vi "Delete Data (Entire Stat Page).vi"(0 "Filepath":path, 11 "Error In":errorcluster) -> (15 "Error Out":errorcluster)   [LabVIEW 2013]
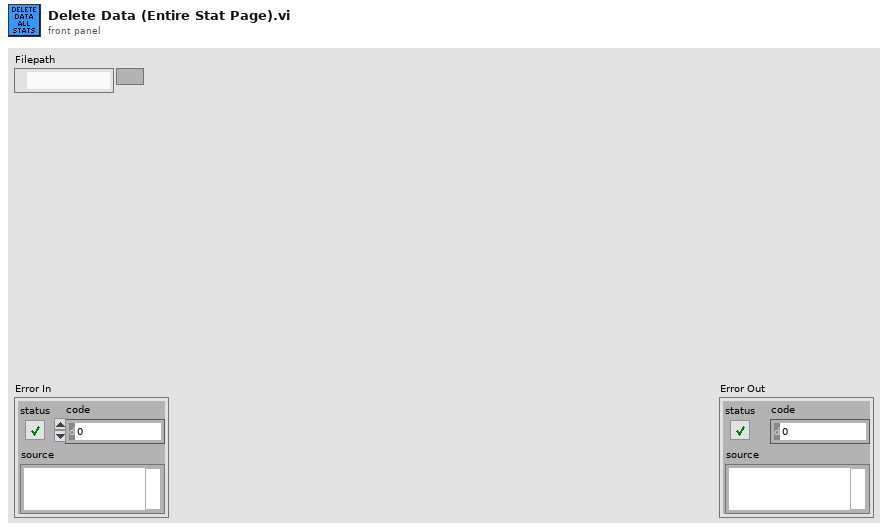
[diagram p1: front panel]
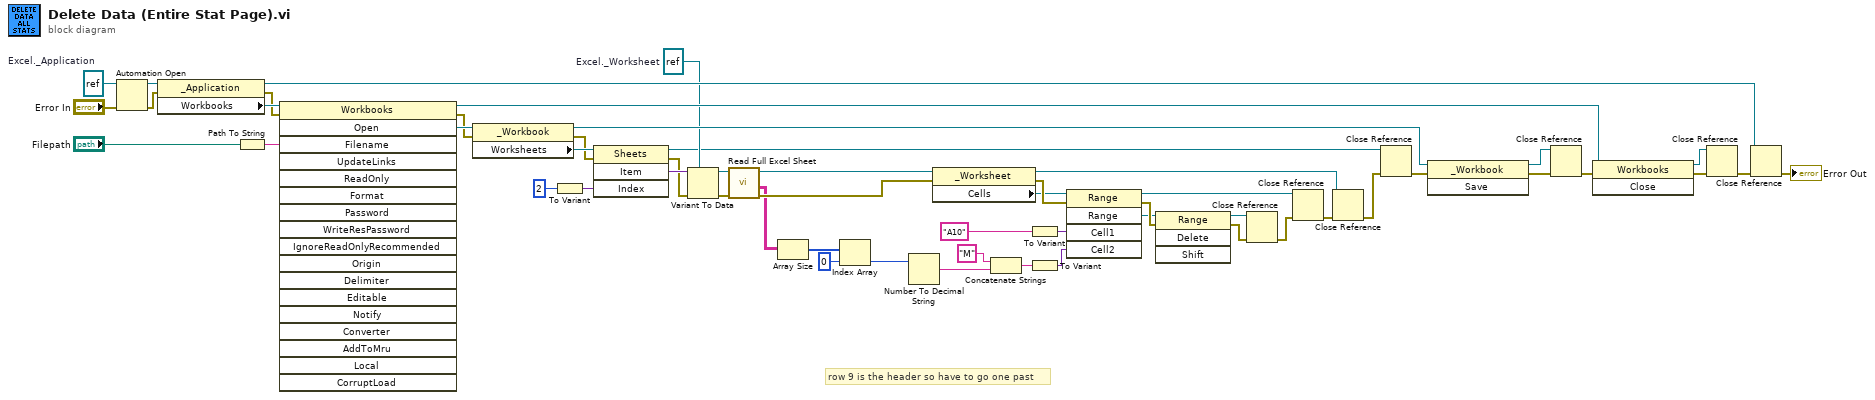
[diagram p0: block diagram]
diagram:
  w18 = refnum<k7> refnum  # Excel._Worksheet
  w51 = refnum<k7> refnum  # Excel._Application
  # "row 9 is the header so have to go one past"
  n1 = Automation Open(error in (no error)="Error In", Automation Refnum=w51) -> (Automation Refnum=w52:refnum<k7>, error out=w53:errorcluster)  [unwired: 2 in]
  n2 = property class="_Application"(reference=w52, error in=w53) -> (reference out=w44:refnum<k7>, error out=w45:errorcluster, "Workbooks"=w54:refnum<k7>)
  n3 = Path To String(path="Filepath") -> (string=w41:string)
  n4 = invoke class="Workbooks" method="Open"(reference=w54, error in=w45, "Filename"=w41) -> (reference out=w48:refnum<k7>, error out=w43:errorcluster, "Open"=w50:refnum<k7>)  [unwired: 15 in, 15 out]
  n5 = property class="_Workbook"(reference=w50, error in=w43) -> (reference out=w37:refnum<k7>, error out=w12:errorcluster, "Worksheets"=w13:refnum<k7>)
  n6 = To Variant(anything=2) -> (Variant=w19:variant)
  n7 = invoke class="Sheets" method="Item"(reference=w13, error in=w12, "Index"=w19) -> (reference out=w17:refnum<k7>, error out=w16:errorcluster, "Item"=w20:variant)  [unwired: 1 in, 1 out]
  n8 = Variant To Data(error in=w16, type=w18, Variant=w20) -> (data=w10:refnum<k7>, error out=w9:errorcluster)
  n9 = call "Read Full Excel Sheet.vi"("Error In"=w9, "Excel._Worksheet"=w10) -> ("Error Out"=w7:errorcluster, "Data"=w6:string[][], "Reference Out"=w8:refnum<k7>)  [unwired: 7 in]
  n10 = Array Size(array=w6) -> (size(s)=w5:i32[])
  n11 = Index Array(array=w5, index=0) -> (element=w3:i32)
  n12 = Number To Decimal String(number=w3) -> (decimal integer string=w14:string)  [unwired: 1 in]
  n13 = property class="_Worksheet"(reference=w8, error in=w7) -> (reference out=w22:refnum<k7>, error out=w26:errorcluster, "Cells"=w25:refnum<k7>)
  n14 = Concatenate Strings("M" ("ColumnIndex"), w14) -> (w32:string)
  n15 = To Variant(anything="A10" ("ColumnIndex")) -> (Variant=w24:variant)
  n16 = To Variant(anything=w32) -> (Variant=w28:variant)
  n17 = invoke class="Range" method="Range"(reference=w25, error in=w26, "Cell1"=w24, "Cell2"=w28) -> (reference out=w11:refnum<k7>, error out=w29:errorcluster, "Range"=w27:refnum<k7>)  [unwired: 1 in, 2 out]
  n18 = invoke class="Range" method="Delete"(reference=w27, error in=w29) -> (reference out=w30:refnum<k7>, error out=w31:errorcluster)  [unwired: 2 in, 2 out]
  n19 = Close Reference(reference=w30, error in (no error)=w31) -> (error out=w1:errorcluster)
  n20 = Close Reference(reference=w11, error in (no error)=w1) -> (error out=w21:errorcluster)
  n21 = Close Reference(reference=w22, error in (no error)=w21) -> (error out=w15:errorcluster)
  n22 = Close Reference(reference=w17, error in (no error)=w15) -> (error out=w42:errorcluster)
  n23 = invoke class="_Workbook" method="Save"(reference=w37, error in=w42) -> (reference out=w38:refnum<k7>, error out=w39:errorcluster)  [unwired: 1 in, 1 out]
  n24 = Close Reference(reference=w38, error in (no error)=w39) -> (error out=w40:errorcluster)
  n25 = invoke class="Workbooks" method="Close"(reference=w48, error in=w40) -> (reference out=w47:refnum<k7>, error out=w46:errorcluster)  [unwired: 1 in, 1 out]
  n26 = Close Reference(reference=w47, error in (no error)=w46) -> (error out=w49:errorcluster)
  n27 = Close Reference(reference=w44, error in (no error)=w49) -> (error out=→"Error Out":errorcluster)
